vi "rp_execute_script.vi"(6 "Variant in":variant, 7 "Shift Pressed?":bool, 8 "error in (no error)":errorcluster, 10 "QD Combo Box Ref":refnum<vi>, 11 "QD Launch VI Ref":refnum<vi>) -> (0 "error out":errorcluster, 4 "Variant out":variant)   [LabVIEW 2019]
doc: "Executes macro scripts to modify panel and diagram objects. \n\nHelp: Type \"?\" in quick drop text then Ctrl-S.\n\nCreated by: Ryan Pacini\n\nDefault Shortcut - [S]"
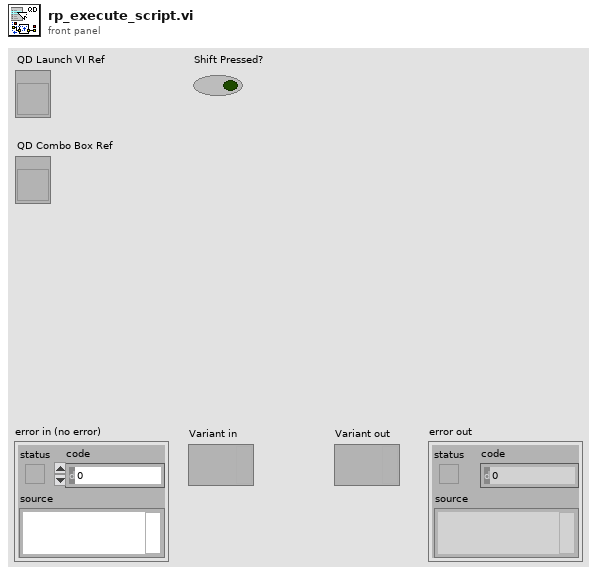
[diagram p1: front panel]
types:
  T1 = typedef "rp_execute_action.ctl" = enum8{"none", "merge_icon", "resize_diagram", "inline_subvi", "open_in_explore", "wire_error_structure", "connect_pane", "arrange_panel_controls", "arrange_panel_indicators", "arrange_diagram_controls", "arrange_diagram_indicators", "align_top_edges", "align_vertical_centers", "align_bottom_edges", "align_left_edges", "align_horizontal_centers", "align_right_edges", "distribute_top_edges", "distribute_vertical_centers", "distribute_bottom_edges", "distribute_vertical_gap", "distribute_vertical_compress", "distribute_left_edges", "distribute_horizontal_centers", "distribute_right_edges", "distribute_horizontal_gap", "distribute_horizontal_compress", "type_u8", "type_u16", "type_u32", "type_u64", "type_i8", "type_i16", "type_i32", "type_i64", "type_sgl", "type_dbl", "type_ext", "type_csg", "type_cdb", "type_cxt", "radix_hide", "radix_dec", "radix_hex", "radix_bin", "inc_dec_hide", "inc_dec_show", "help", "select_controls", "select_indicators", "snap_controls_to_grid", "reset_to_origin"}
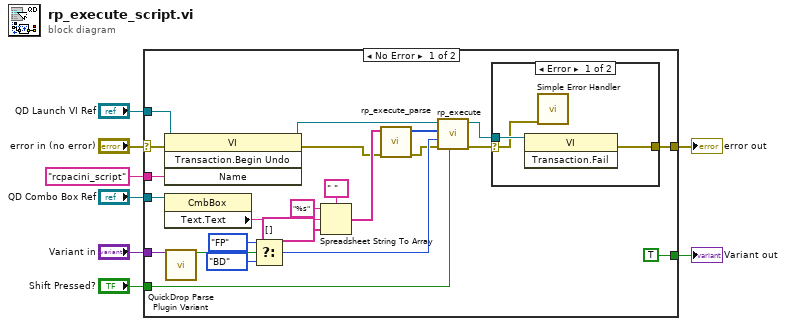
[diagram p0: block diagram]
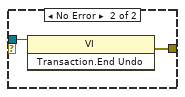
[diagram p2: hidden frame]
diagram:
  n1 = case shown="No Error" "error in (no error)" {
    selector: "error in (no error)" -> [w31 w37]
    tunnel: [w30 w37] -> w4
    tunnel: "QD Launch VI Ref" -> [w27 _]
    tunnel: "rcpacini_script" ("Undo Name") -> [w29 _]
    tunnel: [TRUE _] -> w5
    tunnel: "Variant in" -> [w26 _]
    tunnel: "QD Combo Box Ref" -> [w23 _]
    tunnel: "Shift Pressed?" -> [w18 _]
    frame No Error {
      n2 = invoke class="VI" method="Transaction.Begin Undo"(reference=w27, error in=w31, "Name"=w29) -> (reference out=w25:refnum<vi>, error out=w12:errorcluster)  [unwired: 1 in, 2 out]
      n3 = property class="CmbBox"(reference=w23) -> ("Text.Text"=w9:string)  [unwired: 1 in, 2 out]
      n4 = call <vilib>:"QuickDrop Parse Plugin Variant.vi"("QDKS Variant in"=w26) -> ("QD Launch VI Panel?"=w22:bool)  [unwired: 12 in, 2 out]
      n5 = Select(t=enum8{"FP", "BD"}."FP" ("Panel"), s=w22, f=enum8{"FP", "BD"}."BD" ("Panel")) -> (s? t:f=w19:enum8{"FP", "BD"})
      n6 = Spreadsheet String To Array(delimiter (Tab)=" ", format string="%s", spreadsheet string=w9, array type (2D Dbl)=string[] []) -> (array=w13:string[])
      n7 = call <resource>:"rp_execute_parse.vi"("error in (no error)"=w12, "args"=w13) -> ("error out"=w11:errorcluster, "actions"=w10:T1[])  [unwired: 8 in]
      n8 = call <resource>:"rp_execute.vi"("Shift? (F)"=w18, "error in (no error)"=w11, "Panel"=w19, "actions"=w10, "VI Refnum in"=w25) -> ("error out"=w24:errorcluster, "VI Refnum out"=w17:refnum<vi>)  [unwired: 5 in]
      n9 = case shown="Error" w24 {
        selector: w24 -> [w32 _]
        tunnel: w17 -> [w33 w35]
        tunnel: [w34 w36] -> w30
        frame Error {
          n10 = invoke class="VI" method="Transaction.Fail"(reference=w33) -> (error out=w34:errorcluster)  [unwired: 2 in, 2 out]
          n11 = call <vilib>:"Simple Error Handler.vi"("error in (no error)"=w32) -> ()  [unwired: 4 in, 5 out]
        }
        frame No Error {
          n12 = invoke class="VI" method="Transaction.End Undo"(reference=w35) -> (error out=w36:errorcluster)  [unwired: 2 in, 2 out]
        }
      }
    }
    frame Error {
    }
  }
  "error out" <- w4
  "Variant out" <- w5
